vi "PathPlanner_Trajectory_FindTimeForWaypointRelPos.vi"(9 "WaypointRelPos":dbl, 10 "AllWayPointRelPos":dbl[](array[numeric]), 11 "PathPlannerStates":T1[](array[typedef]) {"TargetHolonomicRotation"."SIN" format="%13.4f"; "TargetHolonomicRotation"."COS" format="%13.4f"; "TargetHolonomicRotation"."VALUE" format="%13.4f"; "Heading"."SIN" format="%13.4f"; "Heading"."COS" format="%13.4f"; "Heading"."VALUE" format="%13.4f"; "PositionMeters"."Y" format="%14.3f"; "PositionMeters"."X" format="%14.3f"}) -> (3 "Time_Secs":dbl)   [LabVIEW 2019, in "PathPlanner24.lvlib"]
doc: "Get the goal state at the given index\n\nIn most (all) cases, using sample() is a better method.\n\nInputs:\n -- Traectory -- PathPlanner Trajectory data cluster\n -- index -- The index of the state to retrieve\n\nOutputs:\n - TrajectoryState -- The state at the given index"
uses:
  TypeDef/PathPlannerTrajectoryState.ctl
  <vilib>/Rock Robotics/WPI/ThirdParty/JAS_Junk/TrajLib/TypeDef/TRANSLATION2D.ctl
  <vilib>/Rock Robotics/WPI/ThirdParty/JAS_Junk/TrajLib/TypeDef/ROTATION2D.ctl
  TypeDef/PathPlannerPathConstraints.ctl
  PathPlanner24.lvlib
  <vilib>/gmath/NI_Gmath.lvlib
  <vilib>/Rock Robotics/WPI/ThirdParty/JAS_Junk/TrajLib/Trajectory_Library.lvlib
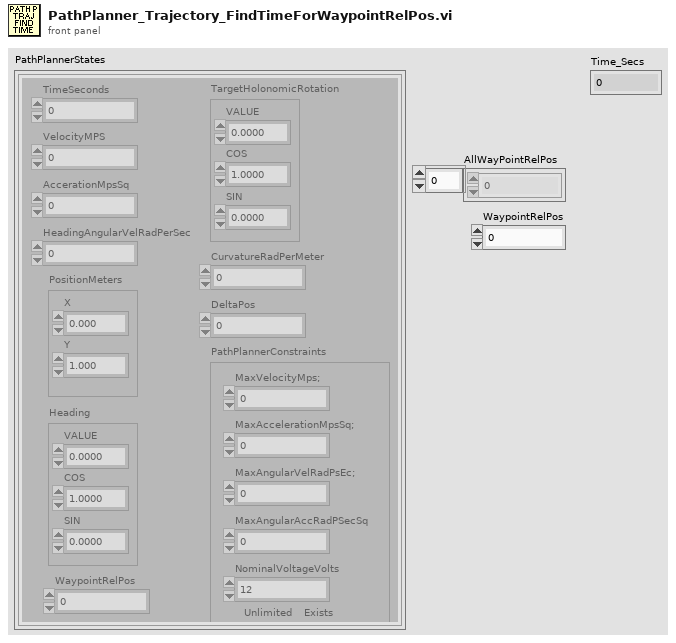
[diagram p1: front panel]
types:
  T1 = typedef "PathPlanner24.lvlib/PathPlannerTrajectoryState.ctl" = cluster{"TimeSeconds":dbl, "VelocityMPS":dbl, "AccerationMpsSq":dbl, "HeadingAngularVelRadPerSec":dbl, "PositionMeters":T2, "Heading":T3, "TargetHolonomicRotation":T3, "CurvatureRadPerMeter":dbl, "PathPlannerConstraints":T4, "DeltaPos":dbl, "WaypointRelPos":dbl}
  T2 = typedef "Trajectory_Library.lvlib/TRANSLATION2D.ctl" = cluster{"X":dbl, "Y":dbl}
  T3 = typedef "Trajectory_Library.lvlib/ROTATION2D.ctl" = cluster{"VALUE":dbl, "COS":dbl, "SIN":dbl}
  T4 = typedef "PathPlanner24.lvlib/PathPlannerPathConstraints.ctl" = cluster{"MaxVelocityMps;":dbl, "MaxAccelerationMpsSq;":dbl, "MaxAngularVelRadPsEc;":dbl, "MaxAngularAccRadPSecSq":dbl, "Exists":bool, "Unlimited":bool, "NominalVoltageVolts":dbl}
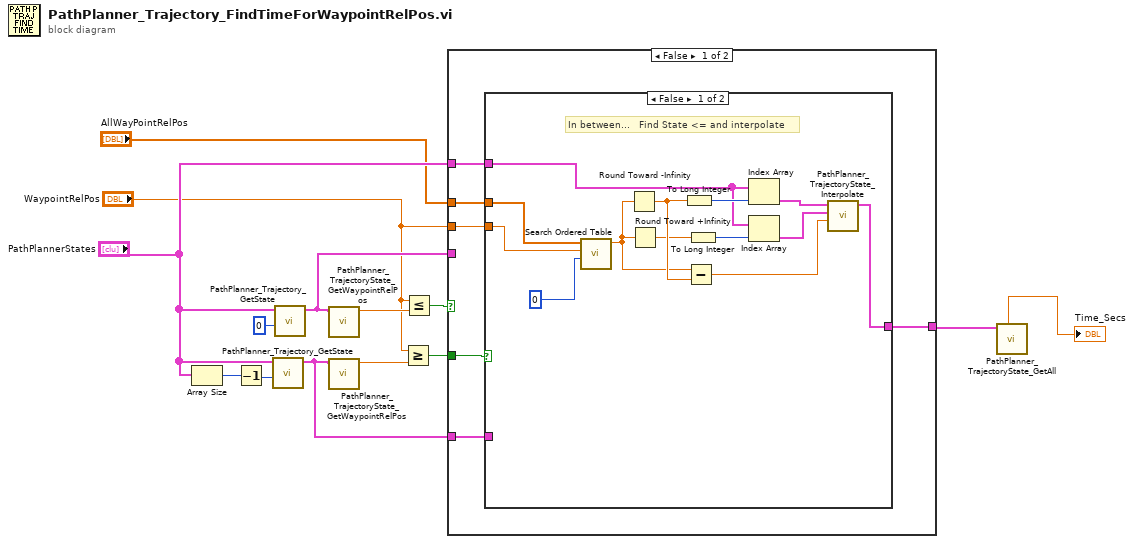
[diagram p0: block diagram]
diagram:
  n1 = Array Size(array="PathPlannerStates") -> (size(s)=w14:i32)
  n2 = Decrement(x=w14) -> (x-1=w13:i32)
  n3 = call "PathPlanner_Trajectory_GetState.vi"("index"=w13, "PathPlannerStates"="PathPlannerStates") -> ("PathPlannerState"=w3:T1)  [unwired: 9 in]
  n4 = call "PathPlanner_Trajectory_GetState.vi"("index"=0, "PathPlannerStates"="PathPlannerStates") -> ("PathPlannerState"=w9:T1)  [unwired: 9 in]
  n5 = call "PathPlanner_TrajectoryState_GetWaypointRelPos.vi"("PathPlannerState"=w9) -> ("WaypointRelPos"=w11:dbl)  [unwired: 10 in]
  n6 = call "PathPlanner_TrajectoryState_GetWaypointRelPos.vi"("PathPlannerState"=w3) -> ("WaypointRelPos"=w6:dbl)  [unwired: 10 in]
  n7 = Greater Or Equal?(x="WaypointRelPos", y=w6) -> (x >= y?=w5:bool)
  n8 = Less Or Equal?(x="WaypointRelPos", y=w11) -> (x <= y?=w10:bool)
  n9 = case shown="False" w10 {
    tunnel: w9 -> [_ w35]
    tunnel: [w18 w35] -> w8
    tunnel: w5 -> [w20 _]
    tunnel: w3 -> [w19 _]
    tunnel: "PathPlannerStates" -> [w17 _]
    tunnel: "AllWayPointRelPos" -> [w16 _]
    tunnel: "WaypointRelPos" -> [w15 _]
    frame False {
      n10 = case shown="False" w20 {
        tunnel: w19 -> [_ w34]
        tunnel: [w21 w34] -> w18
        tunnel: w17 -> [w25 _]
        tunnel: w16 -> [w27 _]
        tunnel: w15 -> [w26 _]
        frame False {
          # "In between...   Find State <= and interpolate"
          n11 = call <vilib>:"Search Ordered Table.vi"("starting index"=0, "x value"=w26, "ordered x array"=w27) -> ("fractional index"=w32:dbl)  [unwired: 8 in]
          n12 = Round Toward -Infinity(1:w32) -> (0:w33:dbl)
          n13 = Round Toward +Infinity(x=w32) -> (ceil(x): smallest int >= x=w31:dbl)
          n14 = To Long Integer(number=w33) -> (32bit integer=w29:i32)
          n15 = Subtract(x=w32, y=w33) -> (x-y=w22:dbl)
          n16 = To Long Integer(number=w31) -> (32bit integer=w30:i32)
          n17 = Index Array(array=w25, index=w29) -> (element=w24:T1)
          n18 = Index Array(array=w25, index=w30) -> (element=w23:T1)
          n19 = call "PathPlanner_TrajectoryState_Interpolate.vi"("Time"=w22, "end Val"=w23, "in PathPlannerState"=w24) -> ("interpolated PathPlanner State"=w21:T1)  [unwired: 8 in]
        }
        frame True {
          # "WaypointPos > last state, use last."
        }
      }
    }
    frame True {
      # "WaypointRelPos <= First State"
    }
  }
  n20 = call "PathPlanner_TrajectoryState_GetAll.vi"("PathPlannerState"=w8) -> ("TimeSeconds"=→"Time_Secs":dbl)  [unwired: 1 in, 9 out]
